vi "GarbageCollect.vi"(8 "Error In":errorcluster) -> (0 "Error Out":errorcluster)   [LabVIEW 2018, in "LabVIEWHTTPClient_NET.lvlib"]
uses:
  LabVIEWHTTPClient_NET.lvlib
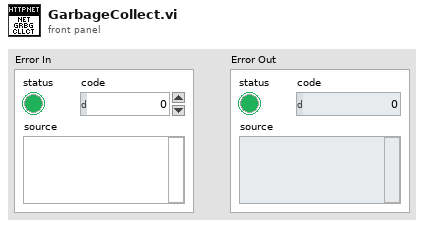
[diagram p1: front panel]
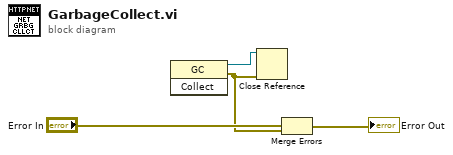
[diagram p0: block diagram]
diagram:
  n1 = invoke class="GC" method="Collect"() -> (reference out=w1:refnum<k24>, error out=w2:errorcluster)  [unwired: 3 in, 1 out]
  n2 = Close Reference(reference=w1, error in (no error)=w2) -> ()  [unwired: 1 out]
  n3 = Merge Errors("Error In", w2) -> (→"Error Out":errorcluster)
